vi "klin1.vi"(6 "Array":i16[](array[numeric])) -> (0 "line":dbl[](array[numeric]), 1 "max отклонение":dbl, 2 "наклон":dbl, 3 "среднее":dbl)   [LabVIEW 2010]
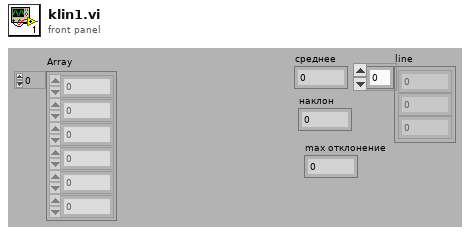
[diagram p1: front panel]
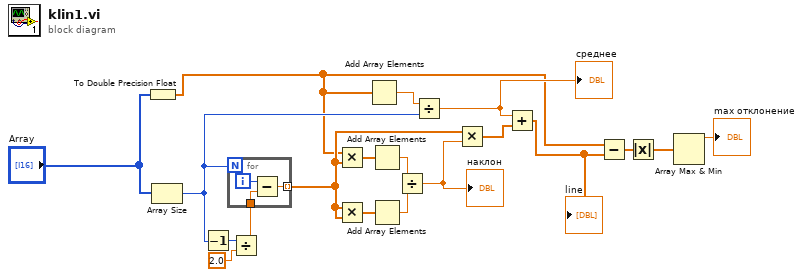
[diagram p0: block diagram]
diagram:
  n1 = To Double Precision Float(number="Array") -> (double precision float=w1:dbl[])
  n2 = Array Size(array="Array") -> (size(s)=w9:i32)
  n3 = Decrement(x=w9) -> (x-1=w10:i32)
  n4 = Divide(x=w10, y=2.0) -> (x/y=w14:dbl)
  n5 = for {
    N: w9 -> [_]
    tunnel: w14 -> [w21]
    tunnel: [w20] -> w4 mode=indexing
    i -> [w22]
    n6 = Subtract(x=w22, y=w21) -> (x-y=w20:dbl)
  }
  n7 = Multiply(x=w1, y=w4) -> (x*y=w17:dbl[])
  n8 = Multiply(x=w4, y=w4) -> (x*y=w18:dbl[])
  n9 = Add Array Elements(numeric array=w1) -> (sum=w13:dbl)
  n10 = Add Array Elements(numeric array=w17) -> (sum=w16:dbl)
  n11 = Add Array Elements(numeric array=w18) -> (sum=w15:dbl)
  n12 = Divide(x=w16, y=w15) -> (x/y=w3:dbl)
  "наклон" <- w3
  n13 = Divide(x=w13, y=w9) -> (x/y=w12:dbl)
  "среднее" <- w12
  n14 = Multiply(x=w4, y=w3) -> (x*y=w11:dbl[])
  n15 = Add(x=w12, y=w11) -> (x+y=w8:dbl[])
  "line" <- w8
  n16 = Subtract(x=w1, y=w8) -> (x-y=w6:dbl[])
  n17 = Absolute Value(x=w6) -> (abs(x)=w7:dbl[])
  n18 = Array Max & Min(array=w7) -> (max value=→"max отклонение":dbl)  [unwired: 3 out]
